vi "Write Config File Ref.vi"(8 "error in (no error)":errorcluster, 10 "refnum in":T1, 11 "Base In":refnum<class "Base.lvclass">) -> (0 "error out":errorcluster, 3 "Base Out":refnum<class "Base.lvclass">)   [LabVIEW 2020, in "Base.lvclass"]
doc: "For the configuration file interface to work, the class implementing the interface needs to save the reference to the file in the class attributes. This is an accessor for that attribute which must be implemented by the class."
uses:
  Base.lvclass
  <vilib>/Utility/config.llb/Config Data RefNum.ctl
  Base.lvclass/Base.ctl
  <vilib>/Utility/config.llb/NI_LVConfig.lvlib
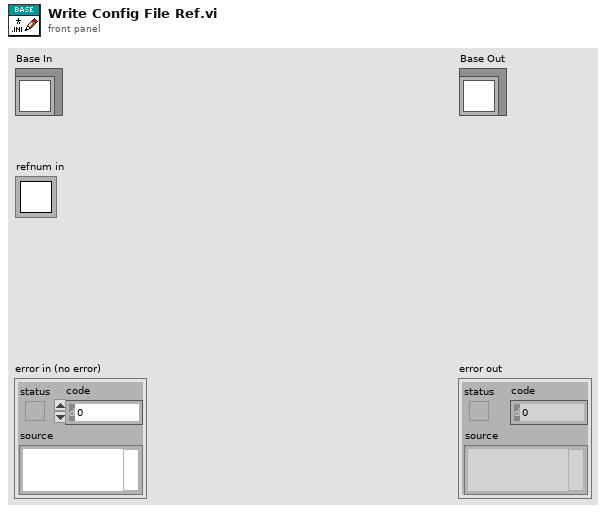
[diagram p1: front panel]
types:
  T1 = typedef "NI_LVConfig.lvlib/Config Data RefNum.ctl" = refnum<k1>
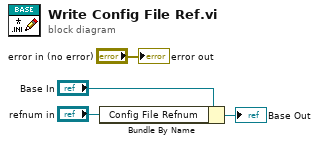
[diagram p0: block diagram]
diagram:
  n1 = Bundle By Name(cluster="Base In", "Config File Refnum"="refnum in") -> (→"Base Out":refnum<class "Base.lvclass">)
  "error out" <- "error in (no error)"
